vi "grSim_RobotReplacement Packet Encoder.vi"(10 "grSim_RobotReplacement":T1) -> (1 "Array":u8[](array[numeric]))   [LabVIEW 2023]
uses:
  grSim RobotReplacement.ctl
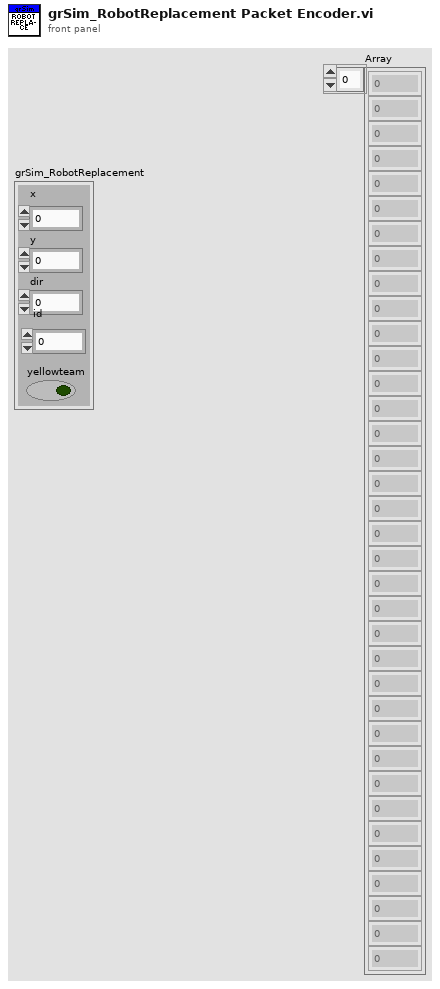
[diagram p1: front panel]
types:
  T1 = typedef "grSim RobotReplacement.ctl" = cluster{"x":dbl, "y":dbl, "dir":dbl, "yellowteam":bool, "id":u32}
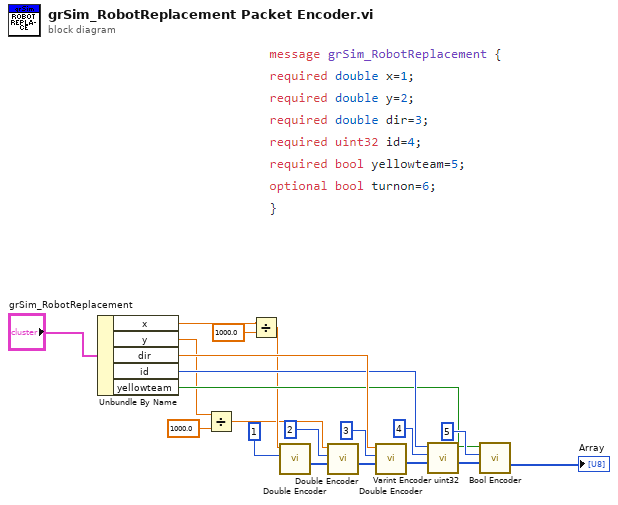
[diagram p0: block diagram]
diagram:
  n1 = Unbundle By Name("grSim_RobotReplacement") -> ("x"=w5:dbl, "y"=w1:dbl, "dir"=w14:dbl, "id"=w11:u32, "yellowteam"=w8:bool)
  n2 = Divide(x=w1, y=1000.0) -> (x/y=w2:dbl)
  n3 = Divide(x=w5, y=1000.0) -> (x/y=w4:dbl)
  n4 = call "Double Encoder.vi"("Key"=u32 1, "Value"=w4) -> ("Array"=w18:u8[])  [unwired: 9 in]
  n5 = call "Double Encoder.vi"("Array In"=w18, "Key"=u32 2, "Value"=w2) -> ("Array"=w17:u8[])  [unwired: 8 in]
  n6 = call "Double Encoder.vi"("Array In"=w17, "Key"=u32 3, "Value"=w14) -> ("Array"=w13:u8[])  [unwired: 8 in]
  n7 = call "Varint Encoder uint32.vi"("Array In"=w13, "Key"=u32 4, "Value"=w11) -> ("Array"=w10:u8[])  [unwired: 8 in]
  n8 = call "Bool Encoder.vi"("Array In"=w10, "Key"=u32 5, "Value"=w8) -> ("Array"=→"Array":u8[])  [unwired: 8 in]
